vi "Authorize.vi"(6 "timeout (ms) [0: default]":i32, 8 "error in (no error)":errorcluster, 10 "State Parameter":string, 11 "Oauth2 in":refnum<class "Oauth2.lvclass">) -> (0 "error out":errorcluster, 2 "Access Token":string, 3 "Oauth2 out":refnum<class "Oauth2.lvclass">)   [LabVIEW 2020, in "Oauth2.lvclass"]
uses:
  Oauth2.lvclass
  Oauth2.lvclass/Oauth2.ctl
  <vilib>/LabVIEW Open Source Project/OpenURI/uri/URI.lvclass/URI.ctl
  OauthClient/OAuthClient.lvclass/OAuthClient.ctl
  <vilib>/LabVIEW Open Source Project/Connection/Connection.TCP/Connection.TCP.lvclass
  C:/Program Files/National Instruments/LabVIEW 2026/vi.lib/LabVIEW Open Source Project/Connection/Connection/Connection.lvclass
  <vilib>/LabVIEW Open Source Project/OpenURI/uri/URI.lvclass
  OAuthToken/OAuth2 Token Element -- enum.ctl
  OAuthToken/OAuthAccessToken.lvclass
  <vilib>/LabVIEW Open Source Project/Connection/Connection/Connection.lvclass
  OauthClient/OAuthClient.lvclass
panel:
  out "Request":string
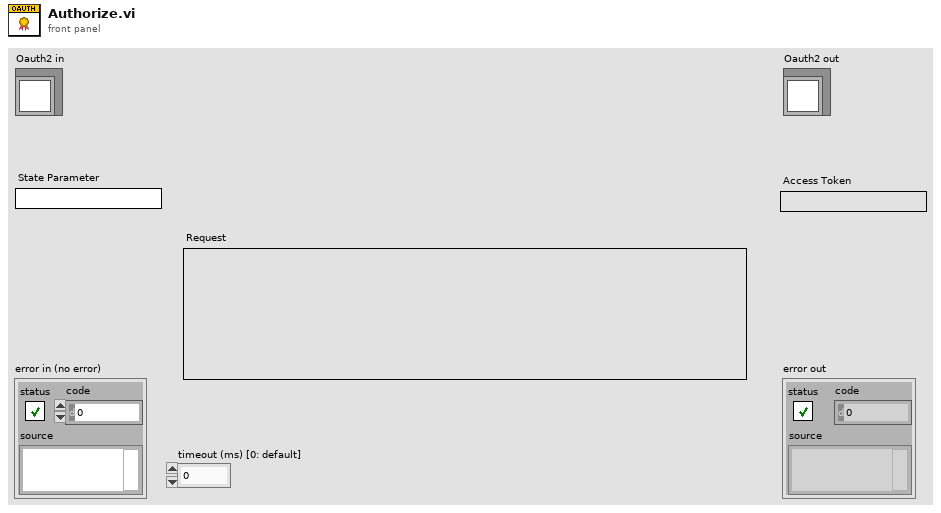
[diagram p1: front panel]
types:
  T1 = typedef "OAuthAccessToken.lvclass/OAuth2 Token Element -- enum.ctl" = enum16{"client_id", "client_secret", "response_type", "scope", "redirect_uri", "error", "error_description", "error_uri", "grant_type", "code", "access_token", "token_type", "expires_in", "username", "password", "refresh_token", "code_challenge", "code_challenge_method", "reverse_proxy_uri", "endpoint element"}
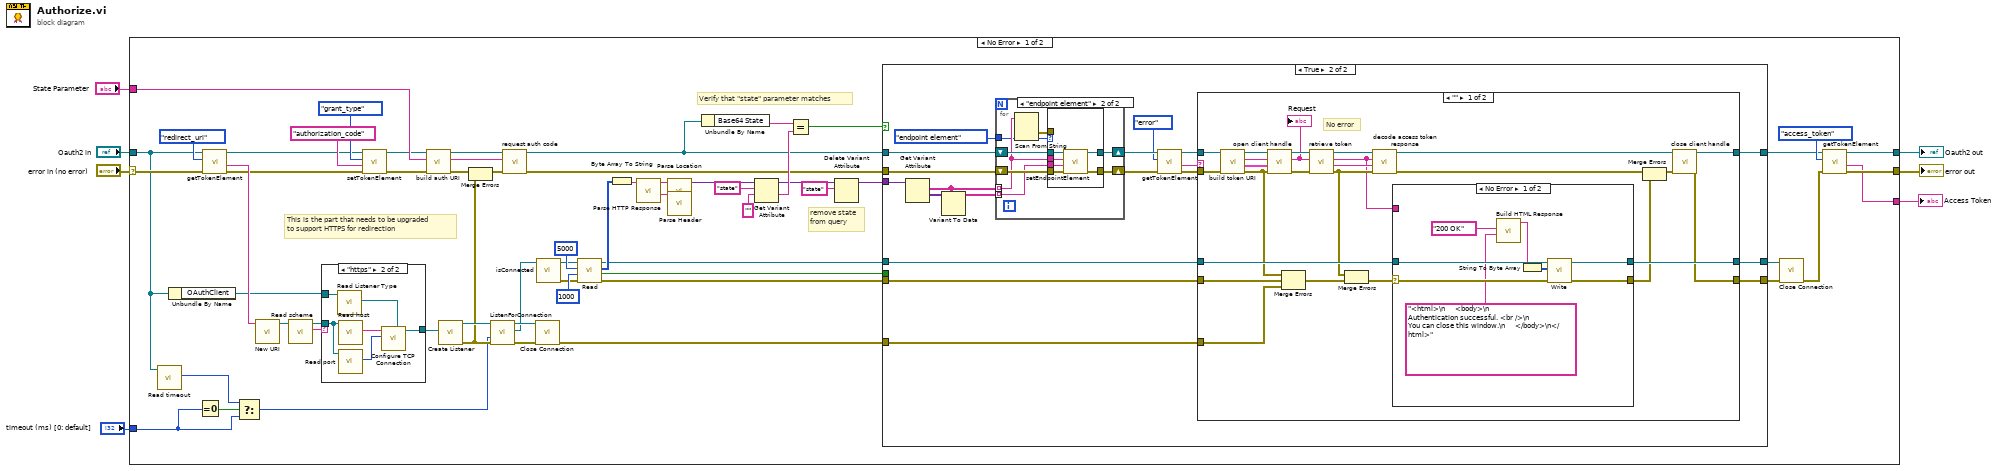
[diagram p0: block diagram]
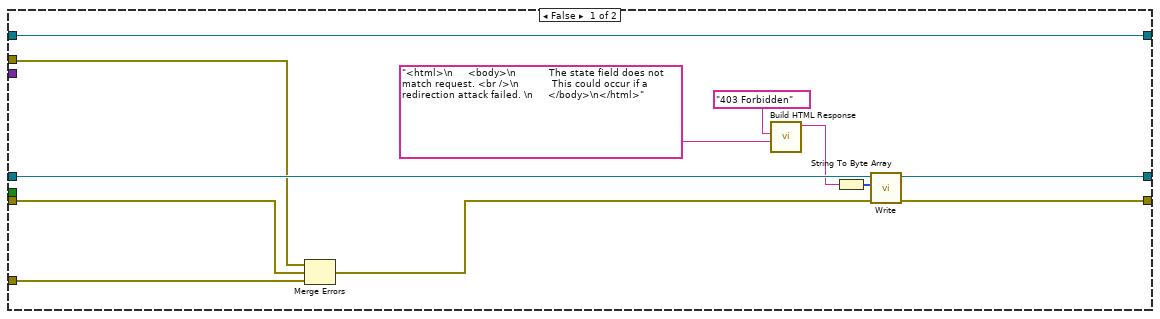
[diagram p2: hidden frame]
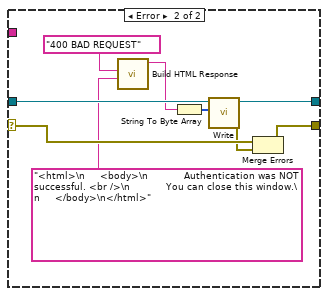
[diagram p3: hidden frame]
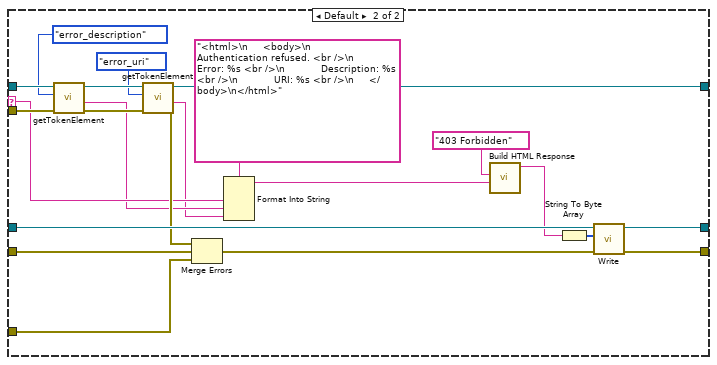
[diagram p4: hidden frame]
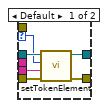
[diagram p5: hidden frame]
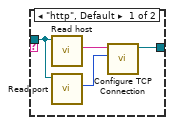
[diagram p6: hidden frame]
diagram:
  n1 = case shown="No Error" "error in (no error)" {
    selector: "error in (no error)" -> [w34 w195]
    tunnel: [w37 w195] -> w6
    tunnel: [w39 w194] -> w4
    tunnel: "Oauth2 in" -> [w9 w194]
    tunnel: "State Parameter" -> [w65 _]
    tunnel: [w30 _] -> w2
    tunnel: "timeout (ms) [0: default]" -> [w13 _]
    frame No Error {
      # "This is the part that needs to be upgraded\nto support HTTPS for redirection"
      # "remove state\nfrom query"
      # "Verify that \"state\" parameter matches"
      n2 = call "Read timeout.vi"("Oauth2 in"=w9) -> ("timeout (ms)"=w11:i32)  [unwired: 8 in, 2 out]
      n3 = Unbundle By Name(w9) -> ("OAuthClient"=w8:refnum<class "OAuthClient.lvclass">)
      n4 = Equal To 0?(x=w13) -> (x = 0?=w45:bool)
      n5 = call "getTokenElement.vi"("error in (no error)"=w34, "Token element"=OAuth2_Token_Element_--_enum."redirect_uri", "Oauth2 in"=w9) -> ("error out"=w12:errorcluster, "Value"=w33:string, "Oauth2 out"=w10:refnum<class "Oauth2.lvclass">)  [unwired: 4 in, 2 out]
      n6 = Select(t=w11, s=w45, f=w13) -> (s? t:f=w44:i32)
      n7 = call <vilib>:"New URI.vi"("URI"=w33) -> ("URI"=w32:refnum<class "URI.lvclass">)  [unwired: 9 in, 1 out]
      n8 = call <vilib>:"Read scheme.vi"("URI in"=w32) -> ("scheme"=w67:string, "URI out"=w66:refnum<class "URI.lvclass">)  [unwired: 8 in, 1 out]
      n9 = case shown="\"https\"" w67 {
        tunnel: w66 -> [w184 w190]
        tunnel: [w185 w191] -> w56
        tunnel: w8 -> [_ w189]
        frame "http", Default {
          n10 = call <vilib>:"Read host.vi"("URI in"=w184) -> ("host"=w187:string)  [unwired: 8 in, 2 out]
          n11 = call <vilib>:"Read port.vi"("URI in"=w184) -> ("port"=w186:u16)  [unwired: 8 in, 2 out]
          n12 = call <vilib>:"Configure TCP Connection.vi"("remote port (80)"=w186, "address (localhost)"=w187) -> ("Connection.TCP"=w185:refnum<class "Connection.TCP.lvclass">)  [unwired: 8 in, 1 out]
        }
        frame "https" {
          n13 = call "Read Listener Type.vi"("OAuthClient in"=w189) -> ("Listener Type"=w188:refnum<class "Connection.TCP.lvclass">)  [unwired: 8 in, 2 out]
          n14 = call <vilib>:"Read host.vi"("URI in"=w190) -> ("host"=w193:string)  [unwired: 8 in, 2 out]
          n15 = call <vilib>:"Read port.vi"("URI in"=w190) -> ("port"=w192:u16)  [unwired: 8 in, 2 out]
          n16 = call <vilib>:"Configure TCP Connection.vi"("Connection.TCP"=w188, "remote port (80)"=w192, "address (localhost)"=w193) -> ("Connection.TCP"=w191:refnum<class "Connection.TCP.lvclass">)  [unwired: 7 in, 1 out]
        }
      }
      n17 = call "setTokenElement.vi"("error in (no error)"=w12, "Value"="authorization_code", "Token element"=OAuth2_Token_Element_--_enum."grant_type", "Oauth2 in"=w10) -> ("error out"=w14:errorcluster, "Oauth2 out"=w15:refnum<class "Oauth2.lvclass">)  [unwired: 6 in]
      n18 = call "build auth URI.vi"("error in (no error)"=w14, "State Parameter"=w65, "Oauth2 in"=w15) -> ("error out"=w50:errorcluster, "Authorization Request URI"=w52:string, "Oauth2"=w51:refnum<class "Oauth2.lvclass">)  [unwired: 6 in]
      n19 = call <vilib>:"Create Listener.vi"("Connection Configuration"=w56) -> ("error out"=w54:errorcluster, "Listener"=w62:refnum<class "Connection.TCP.lvclass">)  [unwired: 9 in]
      n20 = Merge Errors(w50, w54) -> (w53:errorcluster)
      n21 = call <vilib>:"ListenForConnection.vi"("error in (no error)"=w54, "timeout (2000 ms)"=w44, "Listener"=w62) -> ("error out"=w64:errorcluster, "Connection"=w59:refnum<class "Connection.lvclass">, "Listener out"=w61:refnum<class "Connection.TCP.lvclass">)  [unwired: 5 in, 1 out]
      n22 = call-dynamic "request auth code.vi"("error in (no error)"=w53, "Request URI"=w52, "Oauth2 in"=w51) -> ("error out"=w21:errorcluster, "Oauth2 out"=w22:refnum<class "Oauth2.lvclass">)  [unwired: 7 in]
      n23 = call <vilib>:"Close Connection.vi"("error in (no error)"=w64, "Connection in"=w61) -> ("error out"=w47:errorcluster)  [unwired: 8 in, 1 out]
      n24 = call <vilib>:"isConnected.vi"("Connection in"=w59) -> ("error out"=w57:errorcluster, "Connection out"=w58:refnum<class "Connection.lvclass">)  [unwired: 8 in, 1 out]
      n25 = call <vilib>:"Read.vi"("error in (no error)"=w57, "timeout (2000 ms)"=1000 ("bytes to read (100)"), "bytes to read (100)"=5000, "TCPConnection in"=w58) -> ("error out"=w46:errorcluster, "timed out"=w40:bool, "Bytes"=w55:u8[], "TCPConnection out"=w48:refnum<class "Connection.lvclass">)  [unwired: 3 in, 1 out]
      n26 = Byte Array To String(unsigned byte array=w55) -> (string=w29:string)
      n27 = call "Parse HTTP Response.vi"("HTTP Response"=w29) -> ("Header"=w28:string, "Location"=w27:string)  [unwired: 5 in, 4 out]
      n28 = call "Parse Location.vi"("Location"=w27) -> ("Query Parameters"=w26:variant)  [unwired: 10 in]
      n29 = call "Parse Header.vi"("HTTP Header"=w28) -> ()  [unwired: 10 in, 1 out]
      n30 = Unbundle By Name(w22) -> ("Base64 State"=w42:string)
      n31 = Get Variant Attribute(Variant=w26, name="state", default value (empty Variant)="") -> (duplicate Variant=w20:variant, value=w23:string)  [unwired: 1 in, 2 out]
      n32 = Equal?(x=w42, y=w23) -> (x = y?=w41:bool)
      n33 = Delete Variant Attribute(6:"state", 7:w20) -> (3:w19:variant)  [unwired: 1 in, 2 out]
      n34 = case shown="True" w41 {
        tunnel: w22 -> [w72 w92]
        tunnel: w21 -> [w71 w91]
        tunnel: [w77 w98] -> w49
        tunnel: w48 -> [w78 w97]
        tunnel: w47 -> [w75 w96]
        tunnel: w46 -> [w74 w95]
        tunnel: [w72 w94] -> w31
        tunnel: [w76 w93] -> w43
        tunnel: w40 -> [_ _]
        tunnel: w19 -> [_ w86]
        frame False {
          n35 = Merge Errors(w71, w74, w75) -> (w73:errorcluster)
          n36 = call "Build HTML Response.vi"("HTML"="<html>\n     <body>\n           The state field does not match request. <br />\n           This could occur if a redirection attack failed. \n     </body>\n</html>" ("regular expression"), "Status"="403 Forbidden") -> ("HTTP Response"=w68:string)  [unwired: 9 in]
          n37 = String To Byte Array(string=w68) -> (unsigned byte array=w79:u8[])
          n38 = call <vilib>:"Write.vi"("error in (no error)"=w73, "Bytes"=w79, "Connection in"=w78) -> ("error out"=w76:errorcluster, "Connection"=w77:refnum<class "Connection.lvclass">)  [unwired: 7 in]
        }
        frame True {
          n39 = Get Variant Attribute(Variant=w86) -> (names=w87:string[], values=w89:variant[])  [unwired: 3 in, 2 out]
          n40 = Variant To Data(type=w87, Variant=w89) -> (data=w88:string[])  [unwired: 1 in, 1 out]
          n41 = for {
            shift-right: [w169] -> w85
            shift-left: w92 -> [w170]
            shift-right: [w166] -> w83
            shift-left: w91 -> [w168]
            tunnel: w87 -> [w164] mode=indexing
            tunnel: w88 -> [w167] mode=indexing
            tunnel: OAuth2_Token_Element_--_enum."endpoint element" ("Token element") -> [w163]
            n42 = Scan From String(input string=w164, default 1=w163) -> (error out=w165:errorcluster, output 1=w171:T1)  [unwired: 3 in, 2 out]
            n43 = case shown="\"endpoint element\"" w171 {
              selector: w171 -> [w175 _]
              tunnel: w170 -> [w177 w183]
              tunnel: [w176 w182] -> w169
              tunnel: w168 -> [w174 w181]
              tunnel: w167 -> [w173 w179]
              tunnel: [w172 w180] -> w166
              tunnel: w165 -> [_ _]
              tunnel: w164 -> [_ w178]
              frame Default {
                n44 = call "setTokenElement.vi"("error in (no error)"=w174, "Value"=w173, "Token element"=w175, "Oauth2 in"=w177) -> ("error out"=w172:errorcluster, "Oauth2 out"=w176:refnum<class "Oauth2.lvclass">)  [unwired: 6 in]
              }
              frame "endpoint element" {
                n45 = call "setEndpointElement.vi"("error in (no error)"=w181, "Value"=w179, "Endpoint Name"=w178, "Oauth2 in"=w183) -> ("error out"=w180:errorcluster, "Oauth2 out"=w182:refnum<class "Oauth2.lvclass">)  [unwired: 6 in]
              }
            }
          }
          n46 = call "getTokenElement.vi"("error in (no error)"=w83, "Token element"=OAuth2_Token_Element_--_enum."error", "Oauth2 in"=w85) -> ("error out"=w82:errorcluster, "Value"=w80:string, "Oauth2 out"=w84:refnum<class "Oauth2.lvclass">)  [unwired: 4 in, 2 out]
          n47 = case shown="\"\"" w80 {
            selector: w80 -> [_ w147]
            tunnel: [w123 w162] -> w98
            tunnel: w97 -> [w122 w160]
            tunnel: w96 -> [w121 w159]
            tunnel: w95 -> [w120 w158]
            tunnel: [w114 w152] -> w94
            tunnel: [w105 w157] -> w93
            tunnel: w84 -> [w104 w155]
            tunnel: w82 -> [w103 w150]
            frame "" {
              # "No error"
              n48 = call-dynamic "build token URI.vi"("error in (no error)"=w103, "Oauth2 in"=w104) -> ("error out"=w116:errorcluster, "Headers"=w102:cluster{"header":string, "value":string}[], "Token Request URI"=w117:string, "Oauth2"=w118:refnum<class "Oauth2.lvclass">)  [unwired: 6 in]
              n49 = call "open client handle.vi"("error in (no error)"=w116, "Headers"=w102, "Request URI in"=w117, "Oauth2 in"=w118) -> ("error out"=w112:errorcluster, "Request URI dup"=w111:string, "Oauth2 out"=w113:refnum<class "Oauth2.lvclass">)  [unwired: 5 in]
              "Request" <- w111
              n50 = Merge Errors(w116, w120, w121) -> (w119:errorcluster)
              n51 = call "retrieve token.vi"("error in (no error)"=w112, "Token Request URI"=w111, "Oauth2 in"=w113) -> ("error out"=w108:errorcluster, "Response"=w106:string, "Header"=w99:string, "Oauth2 out"=w110:refnum<class "Oauth2.lvclass">)  [unwired: 5 in]
              n52 = Merge Errors(w108, w119) -> (w100:errorcluster)
              n53 = call-dynamic "decode access token response.vi"("error in (no error)"=w108, "Response"=w106, "Header"=w99, "Oauth2 in"=w110) -> ("error out"=w107:errorcluster, "Oauth2"=w109:refnum<class "Oauth2.lvclass">)  [unwired: 6 in]
              n54 = case shown="No Error" w100 {
                selector: w100 -> [w127 w137]
                tunnel: [w131 w140] -> w123
                tunnel: w122 -> [w129 w138]
                tunnel: [w128 w135] -> w101
                tunnel: w99 -> [_ _]
                frame No Error {
                  n55 = call "Build HTML Response.vi"("HTML"="<html>\n     <body>\n            Authentication successful. <br />\n            You can close this window.\n     </body>\n</html>" ("regular expression"), "Status"="200 OK") -> ("HTTP Response"=w125:string)  [unwired: 9 in]
                  n56 = String To Byte Array(string=w125) -> (unsigned byte array=w130:u8[])
                  n57 = call <vilib>:"Write.vi"("error in (no error)"=w127, "Bytes"=w130, "Connection in"=w129) -> ("error out"=w128:errorcluster, "Connection"=w131:refnum<class "Connection.lvclass">)  [unwired: 7 in]
                }
                frame Error {
                  n58 = call "Build HTML Response.vi"("HTML"="<html>\n     <body>\n            Authentication was NOT successful. <br />\n            You can close this window.\n     </body>\n</html>" ("regular expression"), "Status"="400 BAD REQUEST") -> ("HTTP Response"=w132:string)  [unwired: 9 in]
                  n59 = String To Byte Array(string=w132) -> (unsigned byte array=w139:u8[])
                  n60 = call <vilib>:"Write.vi"("Bytes"=w139, "Connection in"=w138) -> ("error out"=w136:errorcluster, "Connection"=w140:refnum<class "Connection.lvclass">)  [unwired: 8 in]
                  n61 = Merge Errors(w137, w136) -> (w135:errorcluster)
                }
              }
              n62 = Merge Errors(w107, w101) -> (w115:errorcluster)
              n63 = call "close client handle.vi"("error in (no error)"=w115, "Oauth2 in"=w109) -> ("error out"=w105:errorcluster, "Oauth2 out"=w114:refnum<class "Oauth2.lvclass">)  [unwired: 8 in]
            }
            frame Default {
              n64 = call "getTokenElement.vi"("error in (no error)"=w150, "Token element"=OAuth2_Token_Element_--_enum."error_description", "Oauth2 in"=w155) -> ("error out"=w151:errorcluster, "Value"=w146:string, "Oauth2 out"=w153:refnum<class "Oauth2.lvclass">)  [unwired: 4 in, 2 out]
              n65 = call "getTokenElement.vi"("error in (no error)"=w151, "Token element"=OAuth2_Token_Element_--_enum."error_uri", "Oauth2 in"=w153) -> ("error out"=w149:errorcluster, "Value"=w145:string, "Oauth2 out"=w152:refnum<class "Oauth2.lvclass">)  [unwired: 4 in, 2 out]
              n66 = Merge Errors(w149, w158, w159) -> (w156:errorcluster)
              n67 = Format Into String(format string="<html>\n     <body>\n            Authentication refused. <br />\n            Error: %s <br />\n            Description: %s <br />\n            URI: %s <br />\n     </body>\n</html>" ("regular expression"), w147, w146, w145) -> (resulting string=w142:string)  [unwired: 2 in, 1 out]
              n68 = call "Build HTML Response.vi"("HTML"=w142, "Status"="403 Forbidden") -> ("HTTP Response"=w141:string)  [unwired: 9 in]
              n69 = String To Byte Array(string=w141) -> (unsigned byte array=w161:u8[])
              n70 = call <vilib>:"Write.vi"("error in (no error)"=w156, "Bytes"=w161, "Connection in"=w160) -> ("error out"=w157:errorcluster, "Connection"=w162:refnum<class "Connection.lvclass">)  [unwired: 7 in]
            }
          }
        }
      }
      n71 = call <vilib>:"Close Connection.vi"("error in (no error)"=w43, "Connection in"=w49) -> ("error out"=w38:errorcluster)  [unwired: 8 in, 1 out]
      n72 = call "getTokenElement.vi"("error in (no error)"=w38, "Token element"=OAuth2_Token_Element_--_enum."access_token", "Oauth2 in"=w31) -> ("error out"=w37:errorcluster, "Value"=w30:string, "Oauth2 out"=w39:refnum<class "Oauth2.lvclass">)  [unwired: 4 in, 2 out]
    }
    frame Error {
    }
  }
  "error out" <- w6
  "Oauth2 out" <- w4
  "Access Token" <- w2
